vi "Global SCALE VIW.vi"() -> ()   [LabVIEW 2019]
panel:
  out "SCALE":T1
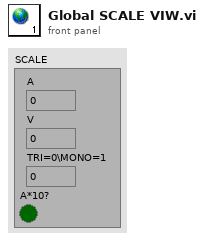
[diagram p1: front panel]
types:
  T1 = cluster{"A":dbl, "V":dbl, "TRI=0\\MONO=1":dbl, "A*10?":bool}
diagram:
